vi "FunctionGenerator_Plot_Example.vi"() -> ()   [LabVIEW 2019]
uses:
  <vilib>/Rock Robotics/WPI/ThirdParty/JAS_Junk/TrajLib/TypeDef/X_Y_PAIR.ctl
  <vilib>/Rock Robotics/WPI/ThirdParty/JAS_Junk/TrajLib/VI/FunctionGenerator_New.vi
  <vilib>/Rock Robotics/WPI/ThirdParty/JAS_Junk/TrajLib/VI/FunctionGenerator_Calculate.vi
  <vilib>/gmath/interp.llb/Search Ordered Table.vi
  <vilib>/Rock Robotics/WPI/ThirdParty/JAS_Junk/TrajLib/Trajectory_Library.lvlib
panel:
  in  "After Entering\nData Pairs Press\nPLOT to plot data":bool
  out "Function Generator":cluster{dbl[], dbl[]}(graph)
  in  "X - Dist Error, Y - Speed Dmd":T1[](array[typedef])=[{"X"=-6.0, "Y"=-2.0}, {"X"=-2.0, "Y"=-2.0}, {"X"=-0.1, "Y"=-0.25}, {"X"=-0.09, "Y"=0.0}, {"X"=0.09, "Y"=0.0}, {"X"=0.1, "Y"=0.25}, {"X"=2.0, "Y"=2.0}, {"X"=6.0, "Y"=2.0}] {"Y" format="%_7f"; "X" format="%_7f"}
  # "Analog  - Function Generator - Example"
  # "Function Generator Example\nThe default values create a function\nthat could be used for position control.\nThe input (x) is position error (Ft).  The output (y)\nis speed demand (Ft/Sec)"
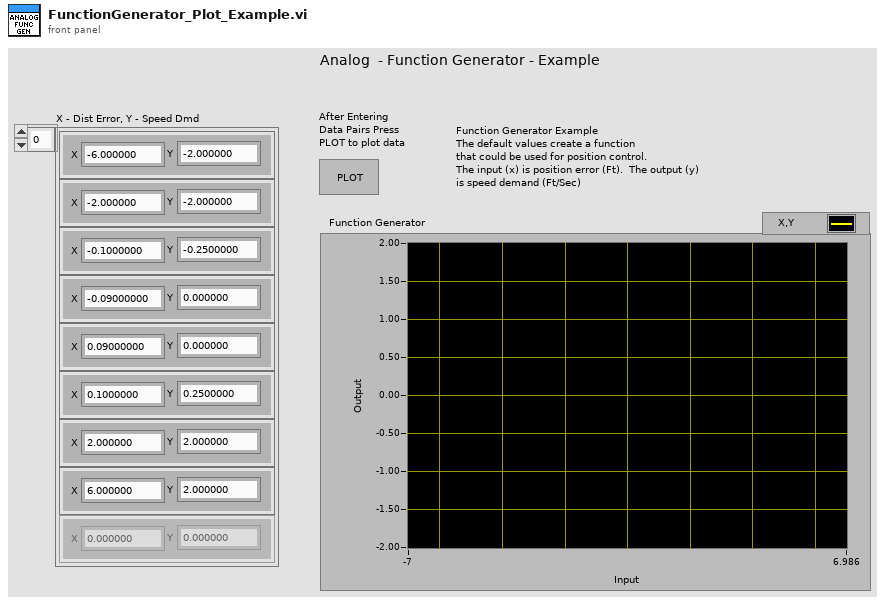
[diagram p1: front panel]
types:
  T1 = typedef "Trajectory_Library.lvlib/X_Y_PAIR.ctl" = cluster{"X":dbl, "Y":dbl}
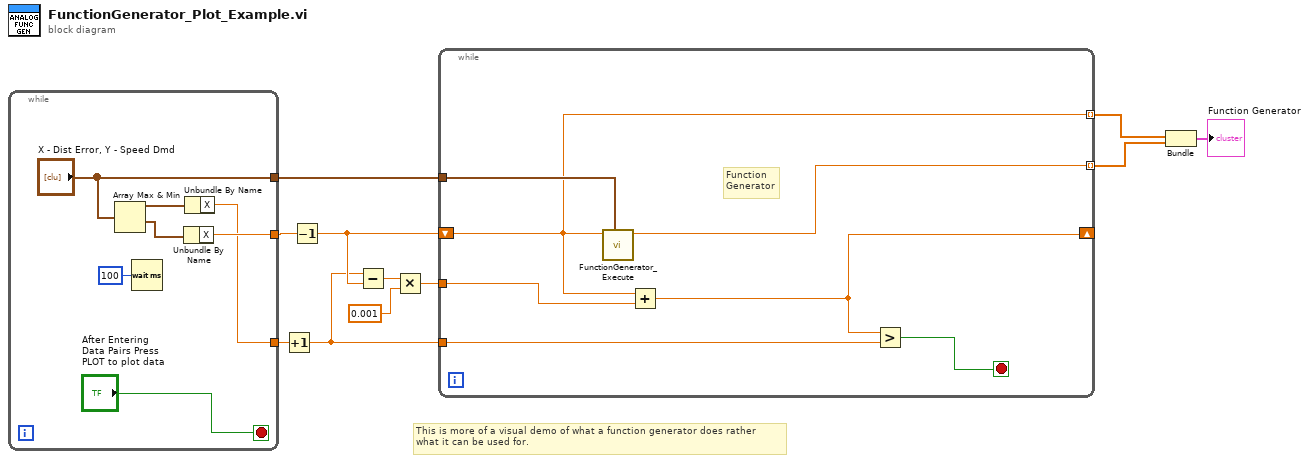
[diagram p0: block diagram]
diagram:
  # "This is more of a visual demo of what a function generator does rather\nwhat it can be used for."
  n1 = while {
    tunnel: ["X - Dist Error, Y - Speed Dmd"] -> w11
    tunnel: [w14] -> w10
    tunnel: [w12] -> w6
    stop <- "After Entering\nData Pairs Press\nPLOT to plot data" stop-if-true
    n2 = Array Max & Min(array="X - Dist Error, Y - Speed Dmd") -> (max value=w13:T1, min value=w15:T1)  [unwired: 2 out]
    n3 = Wait (ms)(milliseconds to wait=u32 100) -> ()  [unwired: 1 out]
    n4 = Unbundle By Name(w15) -> ("X"=w14:dbl)
    n5 = Unbundle By Name(w13) -> ("X"=w12:dbl)
  }
  n6 = Increment(x=w6) -> (x+1=w5:dbl)
  n7 = Decrement(x=w10) -> (x-1=w9:dbl)
  n8 = Subtract(x=w5, y=w9) -> (x-y=w8:dbl)
  n9 = Multiply(x=w8, y=0.001) -> (x*y=w4:dbl)
  n10 = while {
    tunnel: w11 -> [w25]
    shift-right: [w23] -> _
    shift-left: w9 -> [w20]
    tunnel: w5 -> [w22]
    tunnel: w4 -> [w24]
    tunnel: [w20] -> w3 mode=indexing
    tunnel: [w19] -> w2 mode=indexing
    stop <- w21 stop-if-true
    # "Function\nGenerator"
    n11 = call <vilib>:"FunctionGenerator_Execute.vi"("X Y Pairs"=w25, "Input Value"=w20) -> ("Output Value"=w19:dbl)  [unwired: 9 in]
    n12 = Add(x=w20, y=w24) -> (x+y=w23:dbl)
    n13 = Greater?(x=w23, y=w22) -> (0:w21:bool)
  }
  n14 = Bundle(w3, w2) -> (→"Function Generator":cluster{dbl[], dbl[]})  [unwired: 1 in]
